vi "Software Trigger.vi"(8 "error in (no error)":errorcluster, 11 "RP Instrument in":refnum<class "RP Instrument.lvclass">) -> (0 "error out":errorcluster, 3 "RP Instrument out":refnum<class "RP Instrument.lvclass">)   [LabVIEW 2016, in "RP Instrument.lvclass"]
uses:
  RP Instrument.lvclass
  RP Command.ctl
  RP Instrument.lvclass/RP Instrument.ctl
  RP Communicator/RP Communicator.lvclass
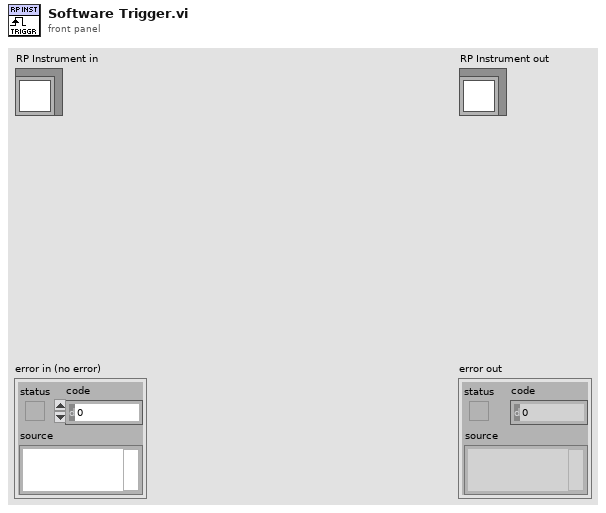
[diagram p1: front panel]
types:
  T1 = typedef "RP Command.ctl" = enum16{"Reset", "Read IDN", "Stop server", "Get status", "Get temperature", "Connect client", "Arm", "Software trigger", "Get whole buffer", "Get chunk", "System call", "Get config", "Set config", "Recieve data", "Play pattern", "Transmit data"}
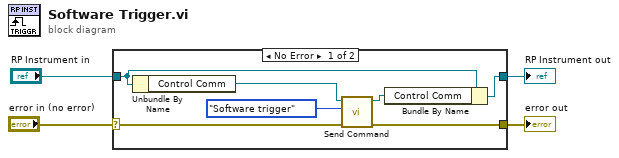
[diagram p0: block diagram]
diagram:
  n1 = case shown="No Error" "error in (no error)" {
    selector: "error in (no error)" -> [w8 w13]
    tunnel: [w7 w13] -> w3
    tunnel: [w6 w12] -> w1
    tunnel: "RP Instrument in" -> [w11 w12]
    frame No Error {
      n2 = Unbundle By Name(w11) -> ("Control Comm"=w10:refnum<class "RP Communicator.lvclass">)
      n3 = call-dynamic "Send Command.vi"("error in (no error)"=w8, "Command number"=RP_Command."Software trigger", "RP Communicator in"=w10) -> ("error out"=w7:errorcluster, "RP Communicator out"=w5:refnum<class "RP Communicator.lvclass">)  [unwired: 7 in]
      n4 = Bundle By Name(cluster=w11, "Control Comm"=w5) -> (w6:refnum<class "RP Instrument.lvclass">)
    }
    frame Error {
    }
  }
  "error out" <- w3
  "RP Instrument out" <- w1
